vi "InitializeVSTForServo.vi"(0 "VSTResourceName":refnum<k15>="RFSG", 11 "error in":errorcluster {"code" format="%.0x"}) -> (4 "powerServoSession":u32, 6 "niRFSGSession":refnum<k15>, 8 "niRFmxInstrSession":refnum<k21>, 10 "niRFSASession":refnum<k15>, 15 "error out":errorcluster)   [LabVIEW 2016, in "Power Servo.lvlib"]
uses:
  Power Servo.lvlib
  <userlib>/_NI Power Servoing IP/HostRdl/NI Power Servoing IP New (Host).lvlib
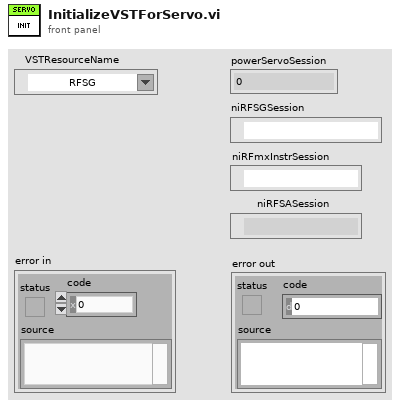
[diagram p1: front panel]
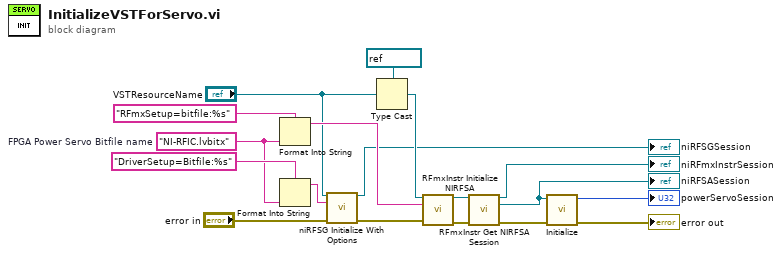
[diagram p0: block diagram]
diagram:
  w14 = "NI-RFIC.lvbitx"  # FPGA Power Servo Bitfile name
  n1 = Format Into String(format string="RFmxSetup=bitfile:%s", w14) -> (resulting string=w15:string)  [unwired: 2 in, 1 out]
  n2 = Format Into String(format string="DriverSetup=Bitfile:%s" ("option string"), w14) -> (resulting string=w17:string)  [unwired: 2 in, 1 out]
  n3 = call <instrlib>:"niRFSG Initialize With Options.vi"("resource name"="VSTResourceName", "option string"=w17, "error in"="error in") -> ("instrument handle"=→"niRFSGSession":refnum<k15>, "error out"=w9:errorcluster)  [unwired: 11 in]
  n4 = Type Cast(type=refnum<k15> "RFSA" ("RFSA Resource Name 2"), x="VSTResourceName") -> (*(type *) &x=w10:refnum<k15>)
  n5 = call <vilib>:"RFmxInstr Initialize NIRFSA.vi"("Resource Name"=w10, "Option String"=w15, "error in (no error)"=w9) -> ("Instrument Handle Out"=w13:refnum<k21>, "error out"=w8:errorcluster)  [unwired: 10 in, 1 out]
  n6 = call <vilib>:"RFmxInstr Get NIRFSA Session.vi"("Instrument Handle In"=w13, "error in (no error)"=w8) -> ("Instrument Handle Out"=→"niRFmxInstrSession":refnum<k21>, "NI RFSA Session"=w4:refnum<k15>, "error out"=w3:errorcluster)  [unwired: 11 in]
  "niRFSASession" <- w4
  n7 = call <userlib>:"Initialize.vi"("error in"=w3, "RFSA Resource Name"=w4) -> ("error out"=→"error out":errorcluster, "SessionHandle"=→"powerServoSession":u32)  [unwired: 8 in]
